vi "Step Execution End.vi"(6 "Skipped":bool, 8 "error in (no error)":errorcluster, 9 "Output Values":cluster{"Name":string, "Variant Data":variant}[](array[cluster]), 10 "Step":refnum<class "Step.lvclass">, 11 "Execution in":refnum<data-value>) -> (0 "error out":errorcluster, 3 "Execution out":refnum<data-value>)   [LabVIEW 2015, in "Execution.lvclass"]
uses:
  Execution.lvclass
  Step.lvclass
  EXECUTION_CTRL_MSG.ctl
  EXECUTION_UI_MSG.ctl
  STEP_END_DATA_TYPEDEF.ctl
  Step/STEP_STATUS.ctl
  STEP_RESULT.ctl
  STEP_MEASURE_RESULT.ctl
  Step/OUTPUT_DATA_TYPE.ctl
  OutputUI/OUTPUT_CHECK_TYPE.ctl
  Send UI Message.vi
  Send Control Message.vi
  Project.lvclass
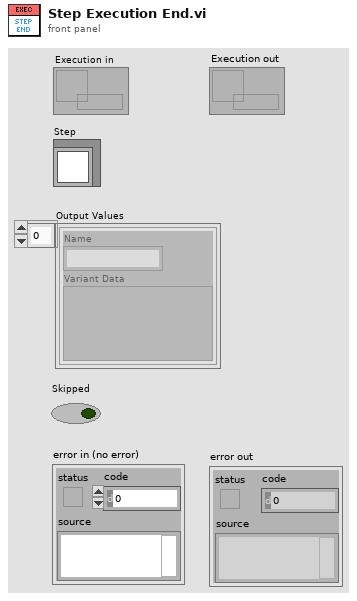
[diagram p1: front panel]
types:
  T1 = typedef "Execution.lvclass/STEP_RESULT.ctl" = cluster{"StepIndex":u32, "Step":refnum<class "Step.lvclass">, "StartTime":timestamp, "EndTime":timestamp, "Result":T2, "Error Info":string, "Measure Results":T3[]}
  T2 = typedef "Step.lvclass/STEP_STATUS.ctl" = enum16{"Skipped", "Done", "Passed", "Failed", "Error"}
  T3 = typedef "Execution.lvclass/STEP_MEASURE_RESULT.ctl" = cluster{"Name":string, "Data Type":T4, "Check Type":T5, "String Limit":string, "Lower Limit":dbl, "Upper Limit":dbl, "Boolean Limit":bool, "Ignore Case":bool, "Measure Data":variant, "Result":T2, "Error Info":string}
  T4 = typedef "Step.lvclass/OUTPUT_DATA_TYPE.ctl" = enum16{"Boolean", "String", "Numeric", "Other"}
  T5 = typedef "Step.lvclass/OUTPUT_CHECK_TYPE.ctl" = enum16{"INVALID", "DO_NOT_CHECK", "RECORD", "VARIABLE", "EQUAL", "NOT_EQUAL", "STR_CONTAINS", "STR_START_WITH", "STR_END_WITH", "STR_REGEX_MATCH", "NUM_GT", "NUM_LT", "NUM_GE", "NUM_LE", "NUM_RANGE", "NUM_RANGE_BDY"}
  T6 = typedef "STEP_END_DATA_TYPEDEF.ctl" = cluster{"Index":i32, "Result":T2, "Duration":dbl, "Value":string, "Low Limit":string, "Upper Limit":string}
  T7 = typedef "Execution.lvclass/EXECUTION_UI_MSG.ctl" = enum16{"EXECUTION_STATUS", "INIT_UI", "DUT_UPDATE", "BOTTOM_PANEL_UPDATE", "TOP_PANEL_UPDATE", "STEP_START", "STEP_END", "DISPLAY_RESULT", "APPLICATION_END"}
  T8 = typedef "Execution.lvclass/EXECUTION_CTRL_MSG.ctl" = enum16{"EXECUTION_START", "EXECUTION_END", "EXECUTION_LOOP", "APPLICATION_STOP"}
  T9 = cluster{"Value":string, "Low Limit":string, "Upper Limit":string}
  T10 = typedef "Execution.lvclass/STEP_CONTEXT.ctl" = cluster{"StepIndex":u32, "Step":refnum<class "Step.lvclass">, "StartTime":timestamp, "EndTime":timestamp, "Result":T2, "Error Info":string, "Output Values":cluster{"Name":string, "Variant Data":variant}[]}
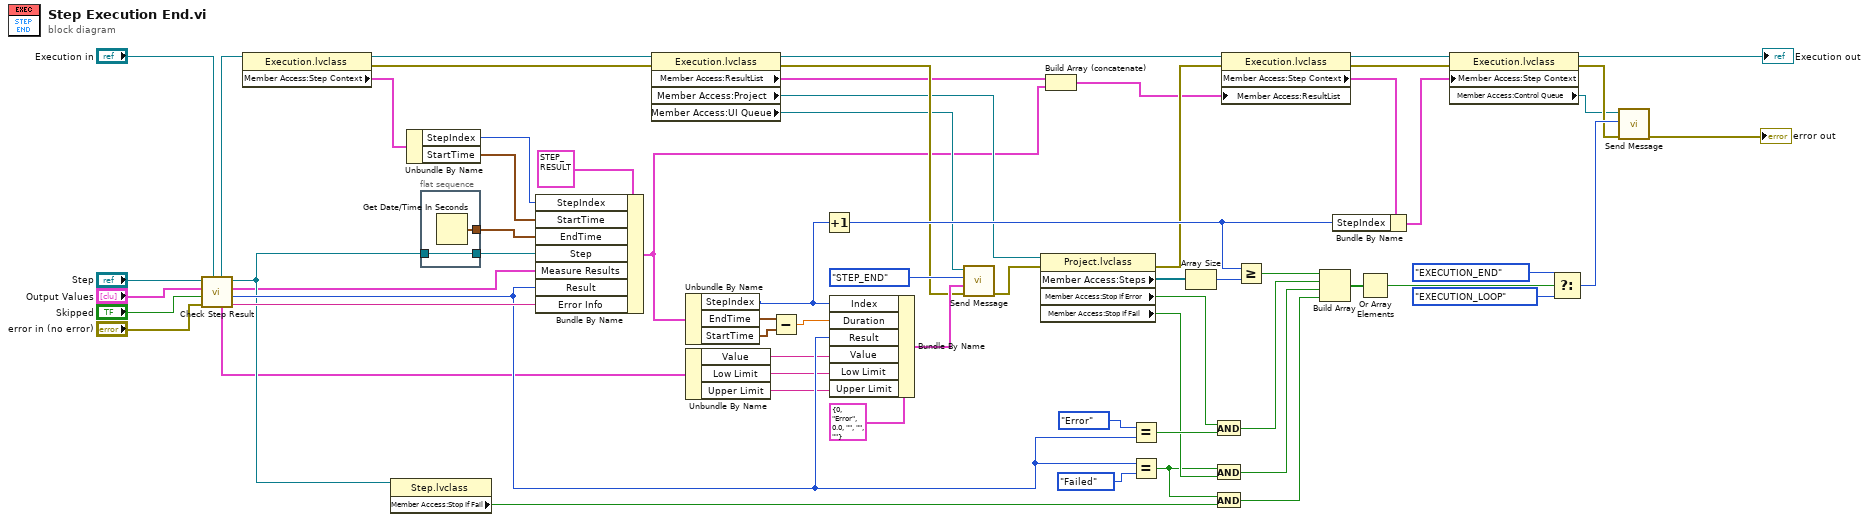
[diagram p0: block diagram]
diagram:
  n1 = call "Check Step Result.vi"("Execution in"="Execution in", "error in (no error)"="error in (no error)", "Skipped"="Skipped", "Output Values in"="Output Values", "Step in"="Step") -> ("Error Info"=w37:string, "Result"=w32:T2, "Measure Results"=w5:T3[], "Step out"=w27:refnum<class "Step.lvclass">, "Value Limit Data"=w4:T9, "Execution out"=w35:refnum<data-value>)  [unwired: 1 in]
  n2 = property class="Execution.lvclass"(reference=w35) -> (reference out=w46:refnum<data-value>, error out=w45:errorcluster, "Member Access:Step Context"=w17:T10)  [unwired: 1 in]
  n3 = property class="Step.lvclass"(reference=w27) -> ("Member Access:Stop If Fail"=w26:bool)  [unwired: 1 in, 2 out]
  n4 = Unbundle By Name(w17) -> ("StepIndex"=w16:u32, "StartTime"=w15:timestamp)
  n5 = flat-sequence {
    tunnel: [w67] -> w50
    tunnel: w27 -> [w66]
    tunnel: [w66] -> w34
    frame #0 {
      n6 = Get Date/Time In Seconds() -> (seconds since 1Jan1904=w67:timestamp)
    }
  }
  n7 = Bundle By Name(cluster=T1 {"StepIndex"=0, "Step"=refnum, "StartTime"=timestamp(0 s since 1904-01-01), "EndTime"=timestamp(0 s since 1904-01-01), "Result"=enum."Error", "Error Info"="", "Measure Results"=[]} ("Step Result"), "StepIndex"=w16, "StartTime"=w15, "EndTime"=w50, "Step"=w34, "Measure Results"=w5, "Result"=w32, "Error Info"=w37) -> (w14:T1)
  n8 = property class="Execution.lvclass"(reference=w46, error in=w45) -> (reference out=w13:refnum<data-value>, error out=w51:errorcluster, "Member Access:ResultList"=w41:T1[], "Member Access:Project"=w42:refnum<class "Project.lvclass">, "Member Access:UI Queue"=w43:refnum<queue>)
  n9 = Unbundle By Name(w14) -> ("StepIndex"=w49:u32, "EndTime"=w48:timestamp, "StartTime"=w47:timestamp)
  n10 = Unbundle By Name(w4) -> ("Value"=w3:string, "Low Limit"=w2:string, "Upper Limit"=w1:string)
  n11 = Subtract(x=w48, y=w47) -> (x-y=w44:dbl)
  n12 = Increment(x=w49) -> (x+1=w57:u32)
  n13 = Bundle By Name(cluster=T6 {"Index"=0, "Result"=enum."Error", "Duration"=0.0, "Value"="", "Low Limit"="", "Upper Limit"=""}, "Index"=w49, "Duration"=w44, "Result"=w32, "Value"=w3, "Low Limit"=w2, "Upper Limit"=w1) -> (w53:T6)
  n14 = call-poly "Send Message.vi"("error in (no error)"=w51, "Data"=w53, "Msg"=EXECUTION_UI_MSG."STEP_END", "UI Queue"=w43) -> ("error out"=w52:errorcluster)  [unwired: 7 in]
  n15 = property class="Project.lvclass"(reference=w42, error in=w52) -> (error out=w10:errorcluster, "Member Access:Steps"=w62:refnum<class "Step.lvclass">[], "Member Access:Stop If Error"=w29:bool, "Member Access:Stop If Fail"=w28:bool)  [unwired: 1 out]
  n16 = Build Array (concatenate)(w41, w14) -> (w9:T1[])
  n17 = Equal?(x=STEP_STATUS."Error" ("Status"), y=w32) -> (x = y?=w30:bool)
  n18 = Equal?(x=w32, y=STEP_STATUS."Failed" ("Status")) -> (x = y?=w25:bool)
  n19 = Array Size(array=w62) -> (size(s)=w61:i32)
  n20 = And(x=w29, y=w30) -> (x .and. y?=w23:bool)
  n21 = And(x=w25, y=w28) -> (x .and. y?=w22:bool)
  n22 = And(x=w25, y=w26) -> (x .and. y?=w21:bool)
  n23 = property class="Execution.lvclass"(reference=w13, error in=w10, "Member Access:ResultList"=w9) -> (reference out=w11:refnum<data-value>, error out=w8:errorcluster, "Member Access:Step Context"=w12:T10)
  n24 = Greater Or Equal?(x=w57, y=w61) -> (x >= y?=w24:bool)
  n25 = Build Array(w24, w23, w22, w21) -> (w20:bool[])
  n26 = Bundle By Name(cluster=w12, "StepIndex"=w57) -> (w7:T10)
  n27 = Or Array Elements(Boolean array=w20) -> (logical OR=w19:bool)
  n28 = property class="Execution.lvclass"(reference=w11, error in=w8, "Member Access:Step Context"=w7) -> (reference out=→"Execution out":refnum<data-value>, error out=w56:errorcluster, "Member Access:Control Queue"=w6:refnum<queue>)
  n29 = Select(t=EXECUTION_CTRL_MSG."EXECUTION_END" ("Msg"), s=w19, f=EXECUTION_CTRL_MSG."EXECUTION_LOOP" ("Msg")) -> (s? t:f=w58:T8)
  n30 = call-poly "Send Message.vi"("error in (no error)"=w56, "Msg"=w58, "Control Queue"=w6) -> ("error out"=→"error out":errorcluster)  [unwired: 8 in]
